vi "PID Plant Identification.vi"(7 "Method":u16(ring) items=["Z-N", "First Order", "S and K", "Second Order"], 8 "Sampling Time":dbl, 9 "with initial part?":bool=TRUE, 10 "Response signal":dbl[](array[numeric]), 11 "Stimulus signal":dbl[](array[numeric])) -> (0 "Time Constant (T) 2":dbl, 1 "Dead Time (L)":dbl, 2 "Time Constant (T)":dbl, 3 "Plant Gain (K)":dbl, 4 "response offset":dbl, 5 "stimulus offset":dbl, 6 "a0":dbl)   [LabVIEW 2017, in "NI_PID_autopid.lvlib"]
uses:
  <vilib>/addons/control/pid/NI_PID_autopid.lvlib
  <vilib>/Analysis/3filter.llb/Filter Passband Type.ctl
  <vilib>/Analysis/1siggen.llb/Ramp Pattern by Delta.vi
  <vilib>/Analysis/3filter.llb/Zero Phase Filter (Cascade, DBL).vi
  <vilib>/Analysis/NI_AALBase.lvlib
  <vilib>/Analysis/NI_AALPro.lvlib
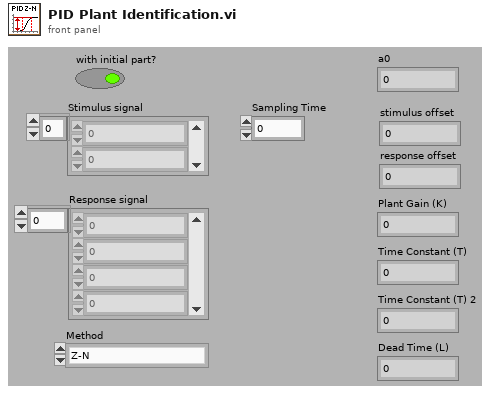
[diagram p1: front panel]
types:
  T1 = typedef "NI_AALBase.lvlib/Filter Passband Type.ctl" = enum32{"Lowpass", "Highpass", "Bandpass", "Bandstop"}
  T2 = cluster{"filter structure":enum32{"IIR 2nd Order", "IIR 4th Order"}, "Reverse Coefficients":dbl[], "Forward Coefficients":dbl[]}
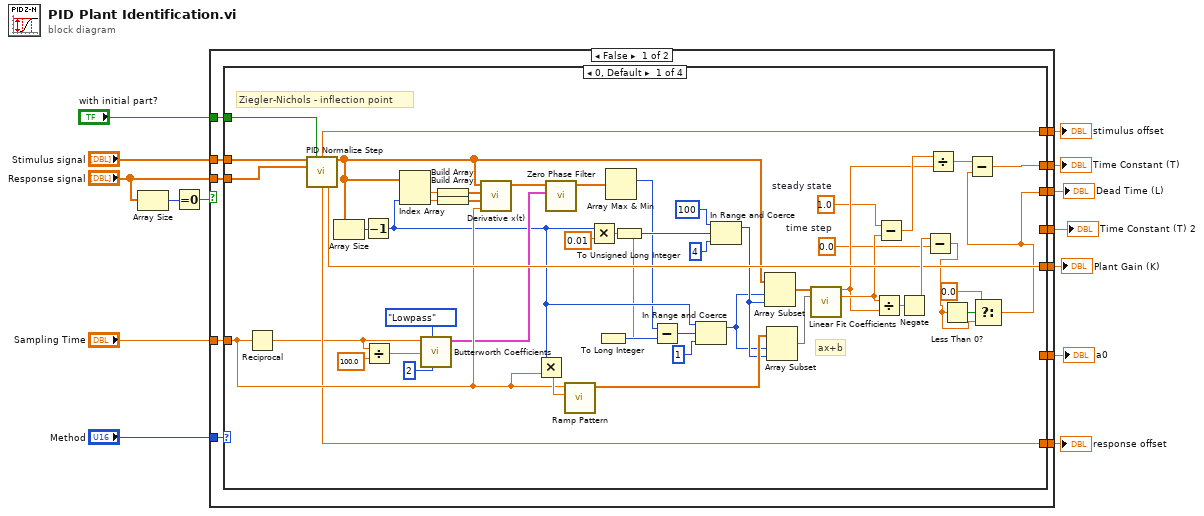
[diagram p0: block diagram]
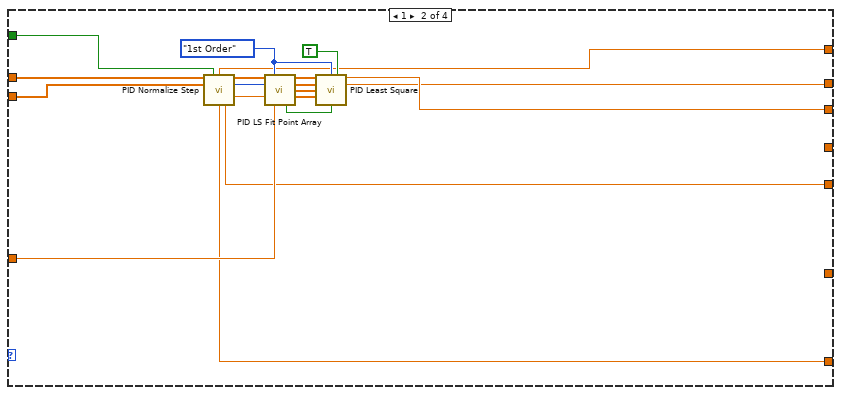
[diagram p2: hidden frame]
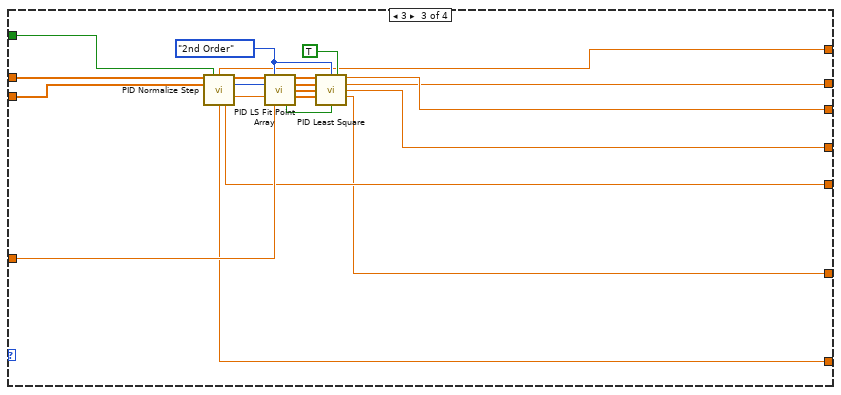
[diagram p3: hidden frame]
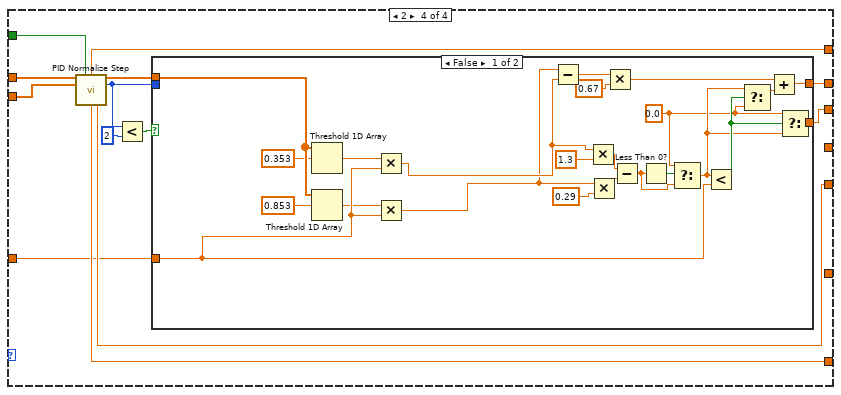
[diagram p4: hidden frame]
diagram:
  n1 = Array Size(array="Response signal") -> (size(s)=w2:i32)
  n2 = Equal To 0?(x=w2) -> (x = 0?=w3:bool)
  n3 = case shown="False" w3 {
    tunnel: [w26 _] -> w14
    tunnel: [w25 _] -> w13
    tunnel: [w24 _] -> w12
    tunnel: "Sampling Time" -> [w23 _]
    tunnel: "Method" -> [w22 _]
    tunnel: [w21 _] -> w9
    tunnel: [w20 _] -> w8
    tunnel: [w19 _] -> w7
    tunnel: [w18 _] -> w6
    tunnel: "Stimulus signal" -> [w17 _]
    tunnel: "Response signal" -> [w16 _]
    tunnel: "with initial part?" -> [w15 _]
    frame False {
      n4 = case shown="0, Default" w22 {
        tunnel: [w71 w81 w102 w122] -> w26
        tunnel: [w70 w80 w101 w129] -> w25
        tunnel: [w42 w82 w103 w121] -> w24
        tunnel: w23 -> [w59 w88 w109 w123]
        tunnel: w17 -> [w48 w90 w111 w127]
        tunnel: w16 -> [w68 w89 w110 w128]
        tunnel: [w53 w79 w100 w124] -> w21
        tunnel: [w52 w78 w99 w125] -> w20
        tunnel: [_ _ w96 _] -> w19
        tunnel: [_ _ w98 _] -> w18
        tunnel: w15 -> [w39 w77 w97 w117]
        frame 0, Default {
          w46 = 1.0  # steady state
          w47 = 0.0  # time step
          # "ax+b"
          # "Ziegler-Nichols - inflection point"
          n5 = Reciprocal(x=w59) -> (1/x=w51:dbl)
          n6 = call <vilib>:"PID Normalize Step.vi"("stimulus signal"=w48, "with initial part?"=w39, "response signal"=w68) -> ("stimulus offset"=w53:dbl, "response norm"=w41:dbl[], "response offset"=w52:dbl, "K"=w70:dbl)  [unwired: 5 in, 4 out]
          n7 = Array Size(array=w41) -> (size(s)=w56:i32)
          n8 = Decrement(x=w56) -> (x-1=w30:i32)
          n9 = Divide(x=w51, y=100.0) -> (x/y=w49:dbl)
          n10 = Index Array(array=w41, index #2=w30) -> (element #1=w58:dbl, element #2=w54:dbl)  [unwired: 1 in]
          n11 = call <vilib>:"Butterworth Coefficients.vi"("order"=2, "filter type"=Filter_Passband_Type."Lowpass", "low cutoff freq: fl"=w49, "sampling freq: fs"=w51) -> ("IIR Filter Cluster"=w38:T2)  [unwired: 6 in, 1 out]
          n12 = Build Array(w58) -> (w57:dbl[])
          n13 = Build Array(w54) -> (w55:dbl[])
          n14 = call <vilib>:"Derivative x(t).vi"("dt"=w59, "Final Condition"=w55, "Initial Condition"=w57, "X"=w41) -> ("dX/dt"=w61:dbl[])  [unwired: 6 in, 1 out]
          n15 = Multiply(x=w30, y=w59) -> (x*y=w76:dbl)
          n16 = call-poly <vilib>:"Zero Phase Filter.vi"("IIR Filter Cluster"=w38, "X"=w61) -> ("Filtered X"=w60:dbl[])  [unwired: 8 in, 1 out]
          n17 = call-poly <vilib>:"Ramp Pattern.vi"("end"=w76, "delta"=w59) -> ("Ramp Pattern"=w69:dbl[])  [unwired: 7 in, 2 out]
          n18 = Multiply(x=w30, y=0.01) -> (x*y=w29:dbl)
          n19 = To Long Integer(number=w29) -> (32bit integer=w31:i32)
          n20 = Array Max & Min(array=w60) -> (max index (indices)=w28:i32)  [unwired: 3 out]
          n21 = To Unsigned Long Integer(number=w29) -> (unsigned 32bit integer=w36:u32)
          n22 = Subtract(x=w28, y=w31) -> (x-y=w27:i32)
          n23 = In Range and Coerce(upper limit=w30, x=w27, lower limit=1) -> (coerced(x)=w32:i32)  [unwired: 1 out]
          n24 = In Range and Coerce(upper limit=u32 100 ("y"), x=w36, lower limit=u32 4 ("y")) -> (coerced(x)=w35:u32)  [unwired: 1 out]
          n25 = Array Subset(array=w41, index=w32, length=w35) -> (w66:dbl[])
          n26 = Array Subset(array=w69, index=w32, length=w35) -> (w67:dbl[])
          n27 = call <vilib>:"Linear Fit Coefficients.vi"("Y"=w66, "X"=w67) -> ("slope"=w64:dbl, "intercept"=w65:dbl)  [unwired: 11 in, 1 out]
          n28 = Divide(x=w65, y=w64) -> (x/y=w75:dbl)
          n29 = Subtract(x=w46, y=w65) -> (x-y=w74:dbl)
          n30 = Negate(x=w75) -> (-x=w72:dbl)
          n31 = Subtract(x=w72, y=w47) -> (x-y=w43:dbl)
          n32 = Divide(x=w74, y=w64) -> (x/y=w73:dbl)
          n33 = Less Than 0?(x=w43) -> (x < 0?=w45:bool)
          n34 = Select(t=0.0, s=w45, f=w43) -> (s? t:f=w42:dbl)
          n35 = Subtract(x=w73, y=w42) -> (x-y=w71:dbl)
        }
        frame 1 {
          w91 = enum16{"1st Order", "2nd Order"}."1st Order" ("TF order")
          n36 = call <vilib>:"PID Normalize Step.vi"("stimulus signal"=w90, "with initial part?"=w77, "response signal"=w89) -> ("stimulus offset"=w79:dbl, "response norm"=w87:dbl[], "length"=w86:i32, "noise"=w85:dbl, "response offset"=w78:dbl, "K"=w80:dbl)  [unwired: 5 in, 2 out]
          n37 = call <vilib>:"PID LS Fit Point Array.vi"("response"=w87, "TF order"=w91, "length"=w86, "noise Band"=w85, "dT"=w88) -> ("double integral delta Y"=w95:dbl[], "integral delta Y"=w94:dbl[], "delta Y at t"=w93:dbl[], "time array"=w92:dbl[], "inverse response"=w84:bool)  [unwired: 6 in]
          n38 = call <vilib>:"PID Least Square.vi"("Double integral delta Y"=w95, "TF order"=w91, "with delay?"=TRUE, "Integral delta Y"=w94, "Delta Y"=w93, "Time array"=w92, "Inverse response?"=w84) -> ("Delay"=w82:dbl, "b1"=w81:dbl)  [unwired: 5 in, 2 out]
        }
        frame 3 {
          w112 = enum16{"1st Order", "2nd Order"}."2nd Order" ("TF order")
          n39 = call <vilib>:"PID Normalize Step.vi"("stimulus signal"=w111, "with initial part?"=w97, "response signal"=w110) -> ("stimulus offset"=w100:dbl, "response norm"=w108:dbl[], "length"=w107:i32, "noise"=w106:dbl, "response offset"=w99:dbl, "K"=w101:dbl)  [unwired: 5 in, 2 out]
          n40 = call <vilib>:"PID LS Fit Point Array.vi"("response"=w108, "TF order"=w112, "length"=w107, "noise Band"=w106, "dT"=w109) -> ("double integral delta Y"=w116:dbl[], "integral delta Y"=w115:dbl[], "delta Y at t"=w114:dbl[], "time array"=w113:dbl[], "inverse response"=w105:bool)  [unwired: 6 in]
          n41 = call <vilib>:"PID Least Square.vi"("Double integral delta Y"=w116, "TF order"=w112, "with delay?"=TRUE, "Integral delta Y"=w115, "Delta Y"=w114, "Time array"=w113, "Inverse response?"=w105) -> ("Delay"=w103:dbl, "b1"=w102:dbl, "b2"=w96:dbl, "a0"=w98:dbl)  [unwired: 5 in]
        }
        frame 2 {
          n42 = call <vilib>:"PID Normalize Step.vi"("stimulus signal"=w127, "with initial part?"=w117, "response signal"=w128) -> ("stimulus offset"=w124:dbl, "response norm"=w126:dbl[], "length"=w120:i32, "response offset"=w125:dbl, "K"=w129:dbl)  [unwired: 5 in, 3 out]
          n43 = Less?(x=w120, y=2) -> (x < y?=w119:bool)
          n44 = case shown="False" w119 {
            tunnel: w126 -> [w135 _]
            tunnel: w120 -> [_ _]
            tunnel: w123 -> [w134 _]
            tunnel: [w143 _] -> w122
            tunnel: [w139 _] -> w121
            frame False {
              w136 = 0.0 ("t")
              n45 = Threshold 1D Array(2:0.353 ("Numeric"), 3:w135) -> (0:w132:dbl)  [unwired: 1 in]
              n46 = Threshold 1D Array(2:0.853 ("Numeric"), 3:w135) -> (0:w131:dbl)  [unwired: 1 in]
              n47 = Multiply(x=w132, y=w134) -> (x*y=w148:dbl)
              n48 = Multiply(x=w131, y=w134) -> (x*y=w147:dbl)
              n49 = Subtract(x=w147, y=w148) -> (x-y=w146:dbl)
              n50 = Multiply(x=w148, y=1.3) -> (x*y=w151:dbl)
              n51 = Multiply(x=w147, y=0.29) -> (x*y=w152:dbl)
              n52 = Multiply(x=w146, y=0.67) -> (x*y=w144:dbl)
              n53 = Subtract(x=w151, y=w152) -> (x-y=w142:dbl)
              n54 = Less Than 0?(x=w142) -> (x < 0?=w141:bool)
              n55 = Select(t=w136, s=w141, f=w142) -> (s? t:f=w137:dbl)
              n56 = Less?(x=w137, y=w134) -> (x < y?=w138:bool)
              n57 = Select(t=w137, s=w138, f=w136) -> (s? t:f=w140:dbl)
              n58 = Add(x=w144, y=w140) -> (x+y=w143:dbl)
              n59 = Select(t=w136, s=w138, f=w137) -> (s? t:f=w139:dbl)
            }
            frame True {
            }
          }
        }
      }
    }
    frame True {
    }
  }
  "Plant Gain (K)" <- w13
  "Dead Time (L)" <- w12
  "Time Constant (T)" <- w14
  "stimulus offset" <- w9
  "response offset" <- w8
  "Time Constant (T) 2" <- w7
  "a0" <- w6
